vi "TEST_Camera_v2.vi"() -> ()   [LabVIEW 2018]
uses:
  <vilib>/vision/Image Controls.llb/IMAQ Image.ctl
  <vilib>/myRIO/Instrument Drivers/Onboard IO/PWM/PWM.lvlib
  <vilib>/vision/driver/NI_Vision_Acquisition_Software.lvlib
  <vilib>/vision/NI_Vision_Development_Module.lvlib
  <vilib>/myRIO/Instrument Drivers/Utilities/Utilities.lvlib
  <vilib>/myRIO/Instrument Drivers/Onboard IO/DIO/DIO.lvlib
  <vilib>/myRIO/Instrument Drivers/Onboard IO/PWM/typedefs/PWM Configuration.ctl
  <vilib>/myRIO/Common/Instrument Driver Framework/myRIO v1.0/PWM/typedefs/PWM Channels Enum.ctl
  <vilib>/myRIO/Common/Instrument Driver Framework/Utilities/typedefs/Generic FPGA Reference.ctl
  <vilib>/myRIO/Common/Instrument Driver Framework/Utilities/typedefs/myRIO v1.0 Reference.ctl
  <vilib>/myRIO/Common/Instrument Driver Framework/Utilities/typedefs/Hardware Version Enum.ctl
  <vilib>/myRIO/Common/Instrument Driver Framework/Utilities/typedefs/myRIO Generic Hardware Reference.ctl
  <vilib>/myRIO/Instrument Drivers/Onboard IO/PWM/typedefs/PWM Reference.ctl
  <vilib>/myRIO/Instrument Drivers/Onboard IO/PWM/vis/myRIO PWM Open.xnode
  <vilib>/myRIO/Common/Instrument Driver Framework/myRIO v1.0/PWM/vis/myRIO v1.1 Open PWM.vi
  <vilib>/userdefined/High Color/nirio_resource_hc.ctl
  <vilib>/myRIO/Instrument Drivers/Onboard IO/UART/typedef/VISA Configuration.ctl
  <vilib>/myRIO/Instrument Drivers/Onboard IO/UART/UART.lvlib
  <vilib>/Instr/_visa.llb/VISA Configure Serial Port (Instr).vi
panel:
  out "error out":errorcluster
  in  "error in (no error)":errorcluster
  out "Character Count":u32
  out "Image 7":T1(plugin-control)
  out "Image Pixels (U8)":u8[][](array[numeric])
  out "Image 6":T1(plugin-control)
  in  "Stop":bool
  out "Image 5":T1(plugin-control)
  out "Y":dbl[](array[numeric])
  out "X":dbl[](array[numeric])
  out "Antal isbjerg":i32
  out "logfile name":path
  in  "logfile base name":string="logfile"
  in  "Color Plane (Color Plane Extraction 1)":i32(ring)=1 items=["Red", "Green", "Blue", "Hue", "Saturation", "Luminance", "Value", "Intensity"]
  in  "Range (Threshold 1)":cluster{"Lower value":sgl, "Upper value":sgl}={"Lower value"=230.0, "Upper value"=255.0}
  in  "Structuring Element (Basic Morphology 1)":i32[][](array[numeric])=[[0, 1, 0], [1, 1, 1], [0, 1, 0]]
  in  "Number of Erosion (Advanced Morphology 1)":i32=12
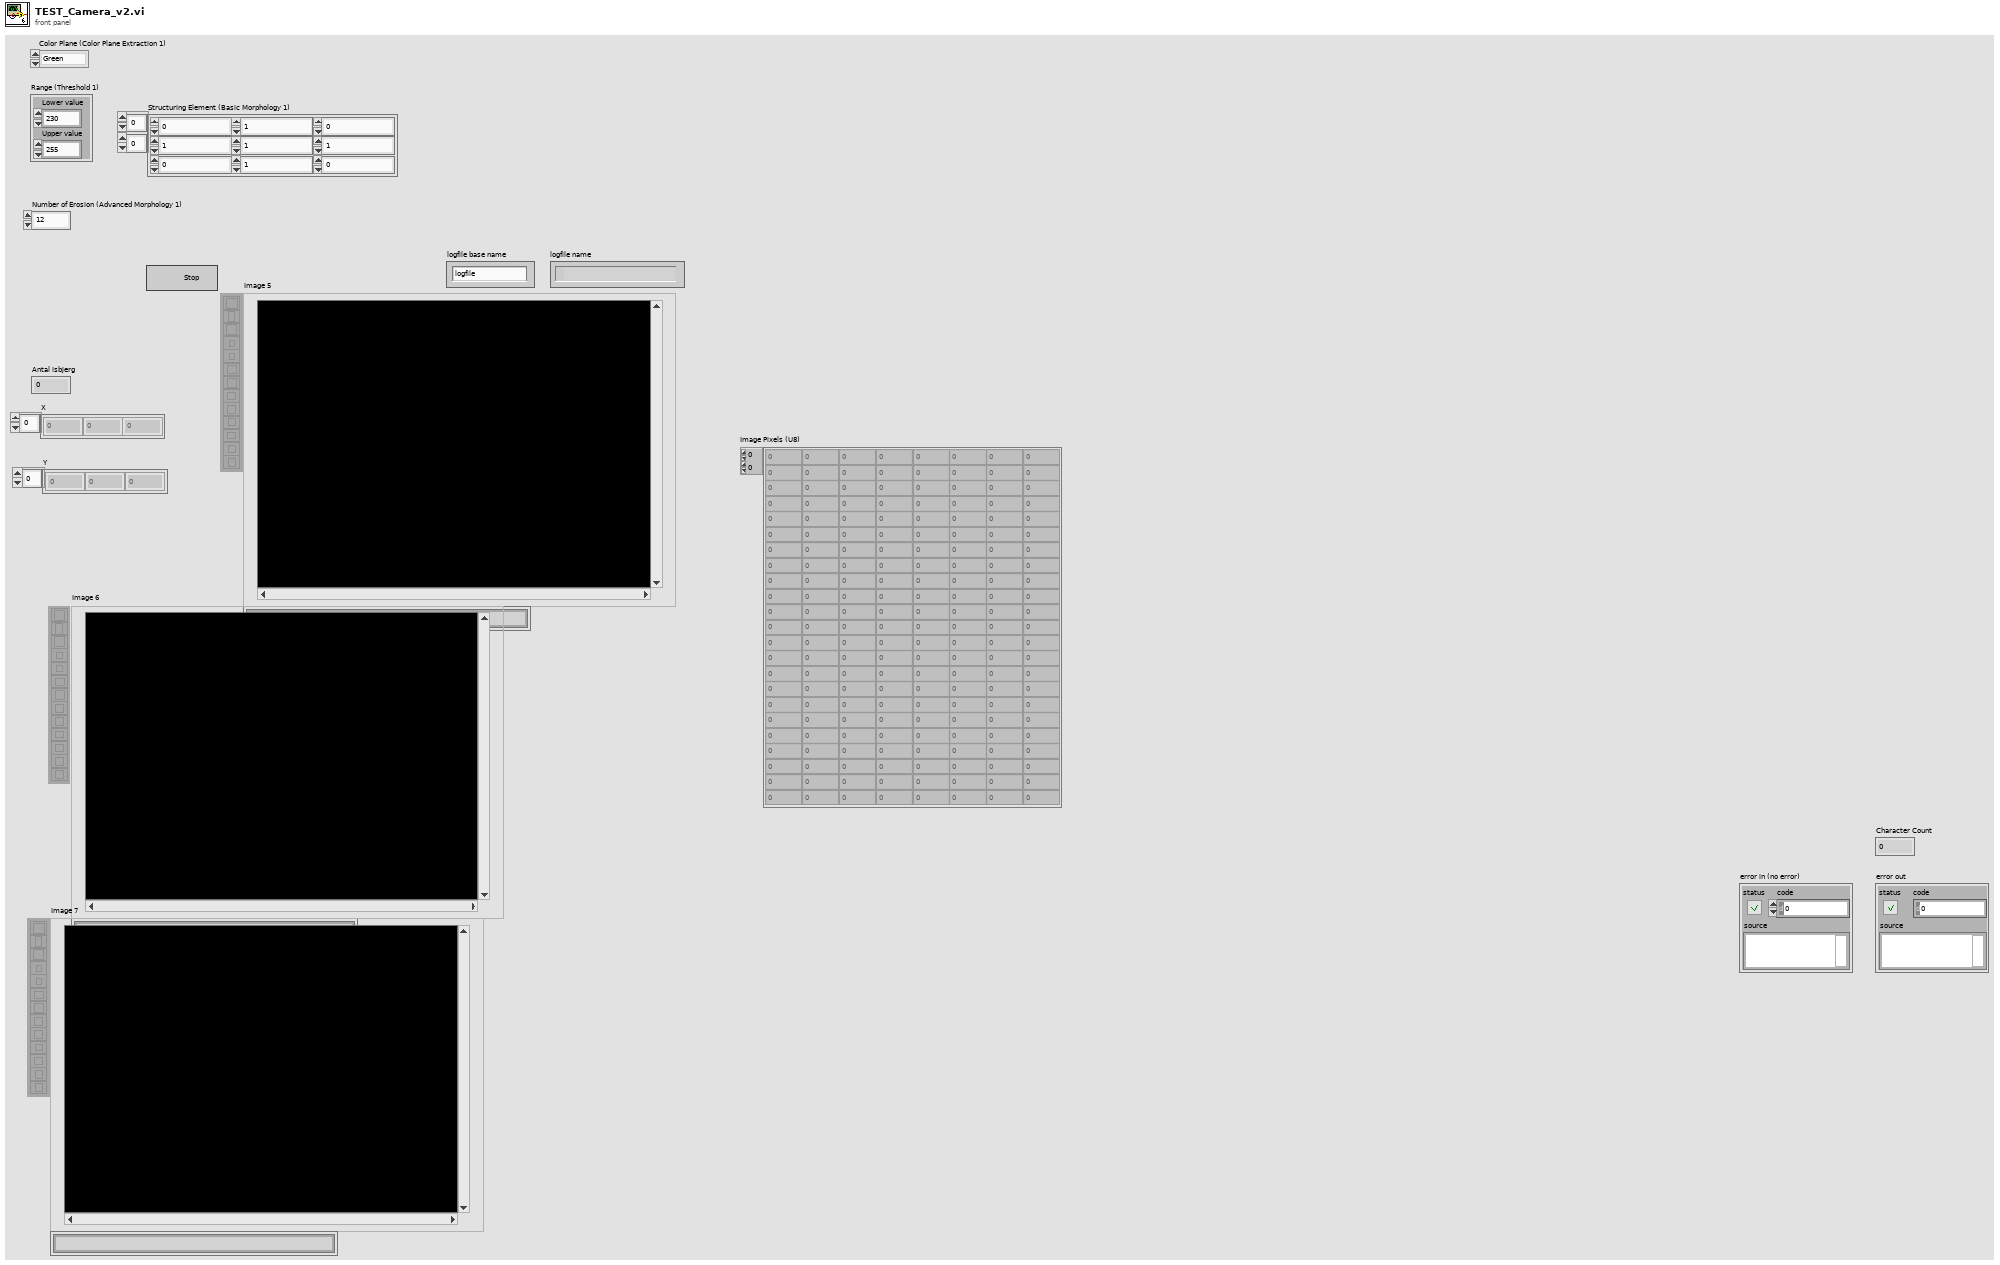
[diagram p1: front panel]
types:
  T1 = typedef "IMAQ Image.ctl" = refnum<image>
  T2 = typedef "UART.lvlib/VISA Configuration.ctl" = cluster{"baud rate (9600)":u32, "data bits (8)":u16, "parity (0:none)":enum16{"None", "Odd", "Even", "Mark", "Space"}, "stop bits (10: 1 bit)":u16, "flow control (0:none)":u16, "termination char\n(0xA = '\\n' = LF) ":u8, "Enable Termination\nChar (T)":bool, "timeout (10sec)":u32}
  T3 = typedef "PWM.lvlib/PWM Reference.ctl" = cluster{"myRIO Reference":T4, "PWM Channels Enum":T8, "PWM Configuration":T9}
  T4 = typedef "myRIO Generic Hardware Reference.ctl" = cluster{"myRIO Model":T5, "myRIO Hardware Reference":T6}
  T5 = typedef "Hardware Version Enum.ctl" = enum16{"Unknown", "myRIO-1900", "myRIO-1950", "roboRIO", "NI ELVIS RIO CM", "ELVIS III"}
  T6 = typedef "myRIO v1.0 Reference.ctl" = cluster{"Generic FPGA Reference":T7, "Allow multiple opens":bool}
  T7 = typedef "Generic FPGA Reference.ctl" = refnum<k20>
  T8 = typedef "PWM Channels Enum.ctl" = enum16{"Not Connected", "C/PWM0", "C/PWM1", "A/PWM0", "A/PWM1", "A/PWM2", "A/PWM3", "A/PWM4", "A/PWM5", "A/PWM6", "A/PWM7", "A/PWM8", "A/PWM9", "A/PWM10", "A/PWM11", "A/PWM12", "A/PWM13", "A/PWM14", "A/PWM15", "A/PWM16", "A/PWM17", "A/PWM18", "A/PWM19", "B/PWM0", "B/PWM1", "B/PWM2", "B/PWM3", "B/PWM4", "B/PWM5", "B/PWM6", "B/PWM7", "B/PWM8", "B/PWM9", "B/PWM10", "B/PWM11", "B/PWM12", "B/PWM13", "B/PWM14", "B/PWM15", "B/PWM16", "B/PWM17", "B/PWM18", "B/PWM19", "PWM/PWM0", "PWM/PWM1", "PWM/PWM2", "PWM/PWM3", "PWM/PWM4", "PWM/PWM5", "PWM/PWM6", "PWM/PWM7", "PWM/PWM8", "PWM/PWM9"}
  T9 = typedef "PWM.lvlib/PWM Configuration.ctl" = cluster{"Frequency":dbl, "Duty Cycle":dbl}
  T10 = enum32{"AutoM", "Close", "Dilate", "Erode", "Gradient", "Gradient out", "Gradient in", "Hit miss", "Open", "PClose", "POpen", "Thick", "Thin"}
  T11 = typedef "Image Type" = u32
  T12 = typedef "IMAQdx.ctl" = refnum<k21>
  T13 = typedef "DIO.lvlib/DIO Reference.ctl" = cluster{"myRIO Reference":T4, "DIO Channels List":T14}
  T14 = typedef "DIO Channels List.ctl" = T15[]
  T15 = typedef "DIO Channels Enum.ctl" = enum16{"Not Connected", "C/DIO0", "C/DIO1", "C/DIO2", "C/DIO3", "C/DIO4", "C/DIO5", "C/DIO6", "C/DIO7", "A/DIO0", "A/DIO1", "A/DIO2", "A/DIO3", "A/DIO4", "A/DIO5", "A/DIO6", "A/DIO7", "A/DIO8", "A/DIO9", "A/DIO10", "A/DIO11", "A/DIO12", "A/DIO13", "A/DIO14", "A/DIO15", "A/DIO16", "A/DIO17", "A/DIO18", "A/DIO19", "B/DIO0", "B/DIO1", "B/DIO2", "B/DIO3", "B/DIO4", "B/DIO5", "B/DIO6", "B/DIO7", "B/DIO8", "B/DIO9", "B/DIO10", "B/DIO11", "B/DIO12", "B/DIO13", "B/DIO14", "B/DIO15", "B/DIO16", "B/DIO17", "B/DIO18", "B/DIO19", "LED0", "LED1", "LED2", "LED3", "Button0", "DIO/DIO0", "DIO/DIO1", "DIO/DIO2", "DIO/DIO3", "DIO/DIO4", "DIO/DIO5", "DIO/DIO6", "DIO/DIO7", "DIO/DIO8", "DIO/DIO9", "SPI/CS0", "SPI/CS1", "SPI/CS2", "SPI/CS3", "LED RADIO (Green)", "LED RADIO (Red)", "LED COMM (Green)", "LED COMM (Red)", "LED MODE (Green)", "LED MODE (Red)"}
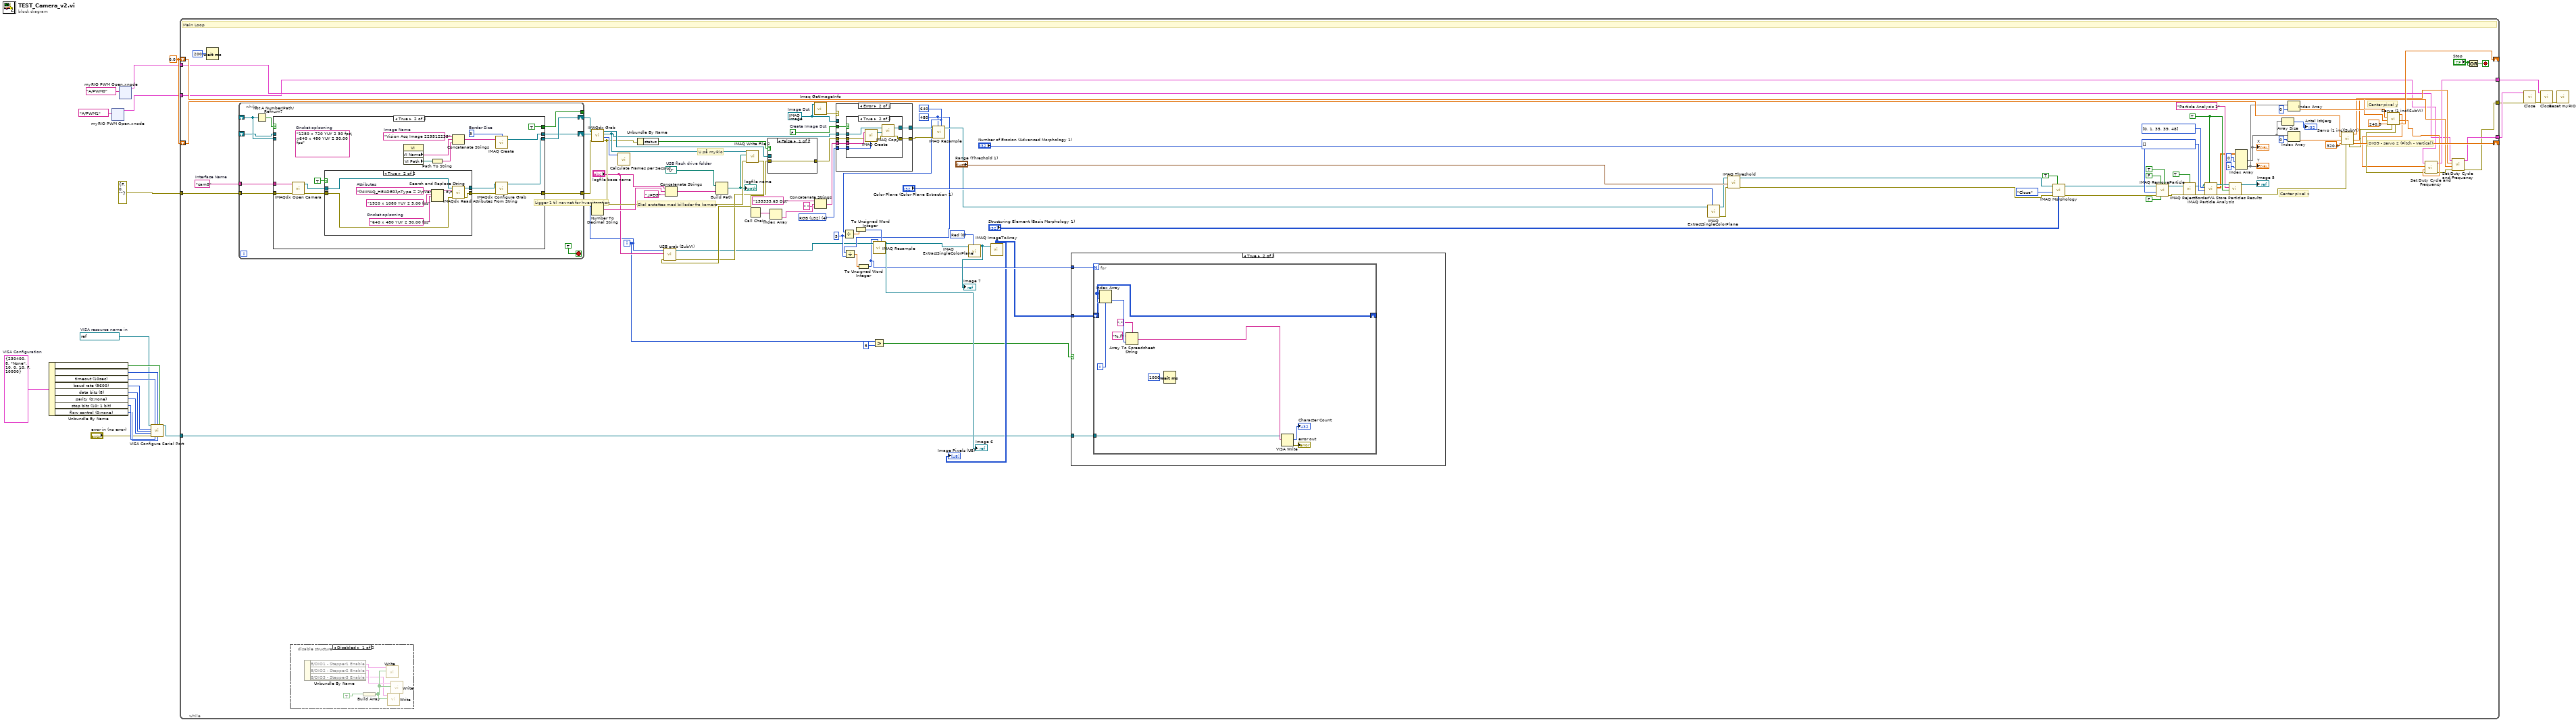
[diagram p0: block diagram]
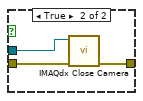
[diagram p4: hidden frame]
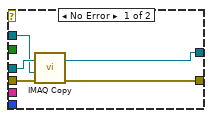
[diagram p7: hidden frame]
diagram:
  w3 = T2 {"baud rate (9600)"=230400, "data bits (8)"=8, "parity (0:none)"=enum."None", "stop bits (10: 1 bit)"=10, "flow control (0:none)"=0, "termination char\n(0xA = '\\n' = LF) "=10, "Enable Termination\nChar (T)"=FALSE, "timeout (10sec)"=10000}  # VISA Configuration
  w2 = refnum<visa-resource-name> "ASRL2::INSTR"  # VISA resource name in
  w22 = 0.0 ("Position 2")
  n1 = Unbundle By Name(w3) -> ("Enable Termination\nChar (T)"=w5:bool, "termination char\n(0xA = '\\n' = LF)"=w6:u8, "timeout (10sec)"=w7:u32, "baud rate (9600)"=w12:u32, "data bits (8)"=w11:u16, "parity (0:none)"=w10:enum16{"None", "Odd", "Even", "Mark", "Space"}, "stop bits (10: 1 bit)"=w9:u16, "flow control (0:none)"=w8:u16)
  n2 = xnode "myRIO PWM Open.xnode"("Channel Name"=tag "A/PWM1") -> ("PWM Ref Out"=w18:T3)  [unwired: 2 in, 1 out]
  n3 = xnode "myRIO PWM Open.xnode"("Channel Name"=tag "A/PWM0") -> ("PWM Ref Out"=w20:T3)  [unwired: 2 in, 1 out]
  n4 = call-poly "VISA Configure Serial Port"("VISA resource name"=w2, "timeout (10sec)"=w7, "termination char\n(0xA = '\\n' = LF)"=w6, "Enable Termination\nChar (T)"=w5, "baud rate (9600)"=w12, "data bits (8)"=w11, "parity (0:none)"=w10, "error in (no error)"="error in (no error)", "stop bits (10: 1 bit)"=w9, "flow control (0:none)"=w8) -> ("VISA resource name out"=w1:refnum<visa-resource-name>)  [unwired: 4 in, 1 out]
  n5 = while {
    shift-right: [w95] -> _
    shift-left: w22 -> [w98]
    shift-right: [w110] -> _
    shift-left: w22 -> [w111]
    tunnel: errorcluster {"status"=FALSE, "code"=0, "source"=""} ("error out") -> [w112]
    tunnel: [w48] -> w15
    tunnel: [w52] -> w16
    tunnel: [w51] -> w17
    tunnel: w20 -> [w31]
    tunnel: w18 -> [w30]
    tunnel: w1 -> [w27]
    i -> [w25]
    stop <- w129 stop-if-true
    w45 = 0 items=["Red", "Green", "Blue", "Hue", "Saturation", "Luminance", "Value", "Intensity"] ("Color Plane")
    w46 = u16 5 ("y")
    w40 = u32 640 ("Width")
    w39 = u32 480 ("Height")
    w67 = i32[] [] items=["Center of Mass X", "Center of Mass Y", "First Pixel X", "First Pixel Y", "Bounding Rect Left", "Bounding Rect Top", "Bounding Rect Right", "Bounding Rect Bottom", "Max Feret Diameter Start X", "Max Feret Diameter Start Y", "Max Feret Diameter End X", "Max Feret Diameter End Y", "Max Horiz. Segment Length Left", "Max Horiz. Segment Length Right", "Max Horiz. Segment Length Row", "-", "Bounding Rect Width", "Bounding Rect Height", "Bounding Rect Diagonal", "Perimeter", "Convex Hull Perimeter", "Holes' Perimeter", "Max Feret Diameter", "Equivalent Ellipse Major Axis", "Equivalent Ellipse Minor Axis", "Equivalent Ellipse Minor Axis (Feret)", "Equivalent Rect Long Side", "Equivalent Rect Short Side", "Equivalent Rect Diagonal", "Equivalent Rect Short Side (Feret)", "Average Horiz. Segment Length", "Average Vert. Segment Length", "Hydraulic Radius", "Waddel Disk Diameter", "-", "Area", "Holes' Area", "Particle & Holes' Area", "Convex Hull Area", "Image Area", "-", "Number of Holes", "Number of Horiz. Segments", "Number of Vert. Segments", "-", "Orientation", "Max Feret Diameter Orientation", "-", "% Area/Image Area", "% Area/(Particle & Holes' Area)", "Ratio of Equivalent Ellipse Axes", "Ratio of Equivalent Rect Sides", "-", "Elongation Factor", "Compactness Factor", "Heywood Circularity Factor", "Type Factor", "-", "Sum X", "Sum Y", "Sum XX", "Sum XY", "Sum YY", "Sum XXX", "Sum XXY", "Sum XYY", "Sum YYY", "-", "Moment of Inertia XX", "Moment of Inertia XY", "Moment of Inertia YY", "Moment of Inertia XXX", "Moment of Inertia XXY", "Moment of Inertia XYY", "Moment of Inertia YYY", "Norm. Moment of Inertia XX", "Norm. Moment of Inertia XY", "Norm. Moment of Inertia YY", "Norm. Moment of Inertia XXX", "Norm. Moment of Inertia XXY", "Norm. Moment of Inertia XYY", "Norm. Moment of Inertia YYY", "Hu Moment 1", "Hu Moment 2", "Hu Moment 3", "Hu Moment 4", "Hu Moment 5", "Hu Moment 6", "Hu Moment 7"] ("Real-World Measurements")
    w68 = i32[] [0, 1, 35, 39, 48] items=["Center of Mass X", "Center of Mass Y", "First Pixel X", "First Pixel Y", "Bounding Rect Left", "Bounding Rect Top", "Bounding Rect Right", "Bounding Rect Bottom", "Max Feret Diameter Start X", "Max Feret Diameter Start Y", "Max Feret Diameter End X", "Max Feret Diameter End Y", "Max Horiz. Segment Length Left", "Max Horiz. Segment Length Right", "Max Horiz. Segment Length Row", "-", "Bounding Rect Width", "Bounding Rect Height", "Bounding Rect Diagonal", "Perimeter", "Convex Hull Perimeter", "Holes' Perimeter", "Max Feret Diameter", "Equivalent Ellipse Major Axis", "Equivalent Ellipse Minor Axis", "Equivalent Ellipse Minor Axis (Feret)", "Equivalent Rect Long Side", "Equivalent Rect Short Side", "Equivalent Rect Diagonal", "Equivalent Rect Short Side (Feret)", "Average Horiz. Segment Length", "Average Vert. Segment Length", "Hydraulic Radius", "Waddel Disk Diameter", "-", "Area", "Holes' Area", "Particle & Holes' Area", "Convex Hull Area", "Image Area", "-", "Number of Holes", "Number of Horiz. Segments", "Number of Vert. Segments", "-", "Orientation", "Max Feret Diameter Orientation", "-", "% Area/Image Area", "% Area/(Particle & Holes' Area)", "Ratio of Equivalent Ellipse Axes", "Ratio of Equivalent Rect Sides", "-", "Elongation Factor", "Compactness Factor", "Heywood Circularity Factor", "Type Factor", "-", "Sum X", "Sum Y", "Sum XX", "Sum XY", "Sum YY", "Sum XXX", "Sum XXY", "Sum XYY", "Sum YYY", "-", "Moment of Inertia XX", "Moment of Inertia XY", "Moment of Inertia YY", "Moment of Inertia XXX", "Moment of Inertia XXY", "Moment of Inertia XYY", "Moment of Inertia YYY", "Norm. Moment of Inertia XX", "Norm. Moment of Inertia XY", "Norm. Moment of Inertia YY", "Norm. Moment of Inertia XXX", "Norm. Moment of Inertia XXY", "Norm. Moment of Inertia XYY", "Norm. Moment of Inertia YYY", "Hu Moment 1", "Hu Moment 2", "Hu Moment 3", "Hu Moment 4", "Hu Moment 5", "Hu Moment 6", "Hu Moment 7"] ("Pixel Measurements")
    w65 = TRUE ("Connectivity 4/8 (8)")
    w88 = path "U:/"  # USB flash drive folder
    w118 = "cam0"  # Interface Name
    w128 = T1 refnum  # Image Dst
    w120 = T11 4 items=["Grayscale (U8)", "Grayscale (I16)", "Grayscale (SGL)", "Complex (CSG)", "RGB (U32)", "HSL (U32)", "RGB (U64)", "Grayscale (U16)"] ("Image Dst Type")
    w126 = FALSE  # Create Image Dst
    # "U på myRio"
    # "Ligger 1 til navnet for hver iteration"
    # "Skal erstattes med billeder fra kamera"
    # "Center pixel y"
    # "Center pixel x"
    # "DIO9 - servo 2 (Pitch - Vertical)"
    # "Main Loop"
    n6 = Wait (ms)(milliseconds to wait=u32 200) -> ()  [unwired: 1 out]
    n7 = while "While Loop_template0" {
      shift-right: [w161] -> w113
      shift-left: _ -> [w154]
      tunnel: [w160] -> w119
      tunnel: w112 -> [w159]
      shift-right: [w157] -> w114
      shift-left: _ -> [w156]
      tunnel: w118 -> [w155]
      tunnel: [w152] -> _
      stop <- TRUE ("_template0") stop-if-true
      n8 = Not A Number/Path/Refnum?(number/path/refnum=w154) -> (NaN/Path/Refnum?=w153:bool)
      n9 = case "Case Structure_template0" shown="True" w153 {
        tunnel: [w164 w180] -> w161
        tunnel: w154 -> [w164 _]
        tunnel: [w163 w179] -> w160
        tunnel: w159 -> [w163 w181]
        tunnel: [w162 w178] -> w157
        tunnel: w156 -> [w162 _]
        tunnel: w155 -> [_ w169]
        tunnel: [_ TRUE] -> w152
        frame False {
        }
        frame True {
          (unwired) "1280 x 720 YUY 2 30 fps\n640 x 480 YUY 2 30.00 fps"  # Ønsket opløsning
          w166 = 3  # Border Size
          w173 = "Vision Acq Image 229512235"  # Image Name
          n10 = call <vilib>:"IMAQdx Open Camera.vi"("error in"=w181, "Session In"=w169) -> ("error out"=w171:errorcluster, "Session Out"=w172:T12)  [unwired: 1 in, 7 out]
          n11 = case shown="True" TRUE ("Init Attributes") {
            tunnel: w172 -> [w183 w191]
            tunnel: w171 -> [w182 w190]
            tunnel: [w183 w189] -> w165
            tunnel: [w182 w188] -> w170
            frame False {
            }
            frame True {
              w184 = "640 x 480 YUY 2 30.00 fps"  # Ønsket opløsning
              w187 = "[NIIMAQ_HEADER]\nType = 2\nVersion = 8\n\n[CAMERA_DATA]\nAcquisitionAttributes::Bayer::Algorithm = \"Bilinear\"\nAcquisitionAttributes::Bayer::GainB = \"1\"\nAcquisitionAttributes::Bayer::GainG = \"1\"\nAcquisitionAttributes::Bayer::GainR = \"1\"\nAcquisitionAttributes::Bayer::Pattern = \"Use hardware value\"\nAcquisitionAttributes::BitsPerPixel = \"Use hardware value\"\nAcquisitionAttributes::HardwareMaximumQueuedBufferCount = \"1000\"\nAcquisitionAttributes::HardwareRequeueBufferListThreshold = \"50\"\nAcquisitionAttributes::IgnoreFirstFrame = \"false\"\nAcquisitionAttributes::ImageDecoderCopyMode = \"Auto\"\nAcquisitionAttributes::OutputImageType = \"Auto\"\nAcquisitionAttributes::OverwriteMode = \"Get Newest\"\nAcquisitionAttributes::PixelSignedness = \"Use hardware value\"\nAcquisitionAttributes::ReceiveTimestampMode = \"None\"\nAcquisitionAttributes::ShiftPixelBits = \"false\"\nAcquisitionAttributes::SwapPixelBytes = \"false\"\nAcquisitionAttributes::Timeout = \"5000\"\nAcquisitionAttributes::VideoMode = \"1920 x 1080 YUY 2 5.00 fps\"\nCameraAttributes::BacklightCompensation::Mode = \"Manual\"\nCameraAttributes::BacklightCompensation::Value = \"0\"\nCameraAttributes::Brightness::Mode = \"Manual\"\nCameraAttributes::Brightness::Value = \"168\"\nCameraAttributes::Contrast::Mode = \"Manual\"\nCameraAttributes::Contrast::Value = \"5\"\nCameraAttributes::Exposure::Mode = \"AutoAperaturePriority\"\nCameraAttributes::Focus::Mode = \"Auto\"\nCameraAttributes::Pan::Mode = \"Manual\"\nCameraAttributes::Pan::Value = \"0\"\nCameraAttributes::PowerLineFrequency::Mode = \"60Hz\"\nCameraAttributes::Saturation::Mode = \"Manual\"\nCameraAttributes::Saturation::Value = \"103\"\nCameraAttributes::Sharpness::Mode = \"Manual\"\nCameraAttributes::Sharpness::Value = \"25\"\nCameraAttributes::Tilt::Mode = \"Manual\"\nCameraAttributes::Tilt::Value = \"0\"\nCameraAttributes::WhiteBalance::Mode = \"Auto\"\nCameraAttributes::Zoom::Mode = \"Manual\"\nCameraAttributes::Zoom::Value = \"0\"\n"  # Attributes
              n12 = Search and Replace String(input string=w187, search string="1920 x 1080 YUY 2 5.00 fps", replace string=w184) -> (result string=w185:string)  [unwired: 5 in, 3 out]
              n13 = call <vilib>:"IMAQdx Read Attributes From String.vi"("error in"=w190, "Attributes String In"=w185, "Session In"=w191) -> ("error out"=w188:errorcluster, "Session Out"=w189:T12)  [unwired: 7 out]
            }
          }
          n14 = property class="VI"() -> ("VI Name"=w176:string, "VI Path"=w177:path)  [unwired: 2 in, 2 out]
          n15 = Path To String(path=w177) -> (string=w175:string)
          n16 = Concatenate Strings(w173, w176, w175) -> (w174:string)
          n17 = call "IMAQ Create"("Border Size"=w166, "Image Name"=w174) -> ("New Image"=w178:T1)  [unwired: 2 in, 2 out]
          n18 = call <vilib>:"IMAQdx Configure Grab.vi"("error in"=w170, "Session In"=w165) -> ("error out"=w179:errorcluster, "Session Out"=w180:T12)  [unwired: 8 out]
        }
      }
    }
    n19 = disable-structure shown="Disabled" {
      frame Disabled {
        n20 = Unbundle By Name() -> ("B/DIO1 - Stepper1 Enable"=w145:T13, "B/DIO2 - Stepper2 Enable"=w144:T13, "B/DIO3 - Stepper3 Enable"=w143:T13)  [unwired: 1 in]
        n21 = Build Array(TRUE) -> (w146:bool[])
        n22 = call <vilib>:"Write.vi"("Values"=w146, "DIO Ref In"=w145) -> ()  [unwired: 7 in, 2 out]
        n23 = call <vilib>:"Write.vi"("Values"=w146, "DIO Ref In"=w143) -> ()  [unwired: 7 in, 2 out]
        n24 = call <vilib>:"Write.vi"("Values"=w146, "DIO Ref In"=w144) -> ()  [unwired: 7 in, 2 out]
      }
      frame Enabled {
      }
    }
    n25 = Number To Decimal String(number=w25) -> (decimal integer string=w91:string)  [unwired: 1 in]
    n26 = call <vilib>:"IMAQdx Grab.vi"("error in"=w119, "Image In"=w114, "Session In"=w113) -> ("error out"=w89:errorcluster, "Buffer Number Out"=w117:u32, "Image Out"=w90:T1, "Session Out"=w116:T12)  [unwired: 1 in, 4 out]
    n27 = call <vilib>:"Calculate Frames per Second.vi"("Buffer Number"=w117) -> ()  [unwired: 2 in, 9 out]
    n28 = Unbundle By Name(w89) -> ("status"=w107:bool)
    n29 = Concatenate Strings "Concatenate Strings"("logfile base name", w91, ".JPEG" ("string")) -> (w36:string)
    n30 = Build Path(base path=w88, name or relative path=w36) -> (appended path=w93:path)
    "logfile name" <- w93
    n31 = call-poly "IMAQ Write File 2"("error in (no error)"=w89, "File Path"=w93, "Image"=w90) -> ("error out"=w34:errorcluster)  [unwired: 7 in, 1 out]
    n32 = call "USB grab (SubVI).vi"("error in (no error)"=w34, "logfile base name in"="logfile base name", "Numeric"=w25) -> ("error out"=w33:errorcluster, "Refnum out"=w32:T1)  [unwired: 7 in]
    n33 = Call Chain() -> (call chain=w125:string[])
    n34 = case "Case Structure_template1" shown="False" w107 {
      tunnel: [w148 w150] -> w115
      tunnel: w33 -> [w148 w151]
      tunnel: w116 -> [_ w149]
      frame False {
      }
      frame True {
        n35 = call <vilib>:"IMAQdx Close Camera.vi"("error in"=w151, "Session In"=w149) -> ("error out"=w150:errorcluster)  [unwired: 9 out]
      }
    }
    n36 = Index Array(array=w125) -> (element=w123:string)  [unwired: 1 in]
    n37 = call "Imaq GetImageInfo"("Image"=w128) -> ("error out"=w127:errorcluster)  [unwired: 1 in, 9 out]
    n38 = Concatenate Strings("155335,63 Dst" ("Image Dst Name"), " ", w123) -> (w121:string)
    n39 = case shown="Error" w127 {
      tunnel: [w196 w200] -> w58
      tunnel: [w195 w199] -> w57
      tunnel: w90 -> [w194 w201]
      tunnel: w115 -> [w193 w197]
      tunnel: w128 -> [w192 _]
      tunnel: w121 -> [_ w203]
      tunnel: w120 -> [_ w202]
      tunnel: w126 -> [_ w198]
      frame No Error {
        n40 = call "IMAQ Copy"("error in (no error)"=w193, "Image Dst"=w192, "Image Src"=w194) -> ("error out"=w195:errorcluster, "Image Dst Out"=w196:T1)  [unwired: 3 out]
      }
      frame Error {
        n41 = case shown="True" w198 {
          tunnel: w203 -> [_ w213]
          tunnel: w202 -> [_ w212]
          tunnel: w201 -> [w205 w210]
          tunnel: [w205 w209] -> w200
          tunnel: [w204 w208] -> w199
          tunnel: w197 -> [w204 w206]
          frame False {
          }
          frame True {
            n42 = call "IMAQ Create"("Image Name"=w213, "Image Type"=w212, "error in (no error)"=w206) -> ("New Image"=w211:T1, "error out"=w207:errorcluster)  [unwired: 1 in, 1 out]
            n43 = call "IMAQ Copy"("error in (no error)"=w207, "Image Dst"=w211, "Image Src"=w210) -> ("error out"=w208:errorcluster, "Image Dst Out"=w209:T1)  [unwired: 3 out]
          }
        }
      }
    }
    n44 = Divide(x=w40, y=w46) -> (x/y=w43:dbl)
    n45 = Divide(x=w39, y=w46) -> (x/y=w44:dbl)
    n46 = To Unsigned Word Integer(number=w43) -> (unsigned 16bit integer=w42:u16)
    n47 = To Unsigned Word Integer(number=w44) -> (unsigned 16bit integer=w29:u16)
    n48 = call "IMAQ Resample"("X Resolution"=w42, "Y Resolution"=w29, "Image Src"=w32) -> ("Image Dst Out"=w38:T1)  [unwired: 7 in, 1 out]
    "Image 6" <- w38
    n49 = Greater?(x=w25, y=5) -> (0:w26:bool)
    n50 = call "IMAQ Resample"("X Resolution"=w40, "Y Resolution"=w39, "error in (no error)"=w57, "Image Src"=w58) -> ("Image Dst Out"=w41:T1)  [unwired: 6 in, 1 out]
    n51 = call "IMAQ ExtractSingleColorPlane"("Color Plane"=w45, "Image Src"=w38) -> ("Image Dst Out"=w37:T1)  [unwired: 8 in, 1 out]
    "Image 7" <- w37
    n52 = call "IMAQ ImageToArray"("Image"=w37) -> ("Image Pixels (U8)"=w28:u8[][])  [unwired: 3 in, 4 out]
    "Image Pixels (U8)" <- w28
    n53 = case shown="True" w26 {
      tunnel: w29 -> [_ w132]
      tunnel: w28 -> [_ w131]
      tunnel: w27 -> [_ w130]
      frame False {
      }
      frame True {
        n54 = for {
          N: w132 -> [_]
          shift-right: [w141] -> _
          shift-left: w131 -> [w141]
          tunnel: w130 -> [w134]
          i -> [w142]
          n55 = Index Array(array=w141, index (row)=w142) -> (element=w140:u8[])  [unwired: 1 in]
          n56 = Array To Spreadsheet String(delimiter (Tab)=",", array=w140, 3:"%.f" ("format string")) -> (spreadsheet string=w135:string)
          n57 = Wait (ms)(milliseconds to wait=u32 1000) -> ()  [unwired: 1 out]
          n58 = VISA Write(VISA resource name=w134, write buffer=w135) -> (return count=→"Character Count":u32, error out=→"error out":errorcluster)  [unwired: 1 in, 1 out]
        }
      }
    }
    n59 = call "IMAQ ExtractSingleColorPlane"("Color Plane"="Color Plane (Color Plane Extraction 1)", "Image Src"=w41) -> ("error out"=w86:errorcluster, "Image Dst Out"=w84:T1)  [unwired: 2 in, 6 out]
    n60 = call "IMAQ Threshold"("error in (no error)"=w86, "Range"="Range (Threshold 1)", "Image Src"=w84) -> ("error out"=w83:errorcluster, "Image Dst Out"=w79:T1)  [unwired: 3 in, 4 out]
    n61 = call "IMAQ Morphology"("Structuring Element"="Structuring Element (Basic Morphology 1)", "Square/Hexa (Square)"=TRUE, "error in (no error)"=w83, "Operation"=T10."Close", "Image Src"=w79) -> ("error out"=w78:errorcluster, "Image Dst Out"=w73:T1)  [unwired: 2 in, 3 out]
    n62 = call "IMAQ RemoveParticle"("Connectivity 4/8 (8)"=TRUE, "Low Pass/High Pass (Low)"=FALSE, "Square/Hexa (Square)"=FALSE, "error in (no error)"=w78, "Number of Erosion"="Number of Erosion (Advanced Morphology 1)", "Image Src"=w73) -> ("error out"=w72:errorcluster, "Image Dst Out"=w70:T1)  [unwired: 1 in, 3 out]
    n63 = call "IMAQ RejectBorder"("error in (no error)"=w72, "Image Src"=w70, "Connectivity 4/8 (8)"=TRUE) -> ("error out"=w69:errorcluster, "Image Dst Out"=w66:T1)  [unwired: 1 in, 2 out]
    n64 = call "IMAQ Particle Analysis"("Connectivity 4/8 (8)"=w65, "error in (no error)"=w69, "Real-World Measurements"=w67, "Pixel Measurements"=w68, "Image"=w66) -> ("error out"=w62:errorcluster, "Particle Measurements (Pixels)"=w59:dbl[][], "Image Out (duplicate)"=w64:T1)  [unwired: 4 out]
    n65 = call <vilib>:"IVA Store Particles Results.vi"("error in (no error)"=w62, "Connectivity 4/8 (8)"=w65, "Step Name"="Particle Analysis 1", "Image in"=w64) -> ("error out"=w60:errorcluster, "Image dup"=→"Image 5":T1)  [unwired: 6 out]
    n66 = Index Array(array=w59, index (col) #1=0 ("index (col)"), index (col) #2=1 ("index (col)")) -> (element #1=w102:dbl[], element #2=w99:dbl[])  [unwired: 2 in]
    "Y" <- w99
    "X" <- w102
    n67 = Array Size(array=w102) -> (size(s)=→"Antal isbjerg":i32)
    n68 = Index Array(array=w99, index=0) -> (element=w94:dbl)
    n69 = Index Array(array=w102, index=0) -> (element=w101:dbl)
    n70 = call "Servo (1 inc)(SubVI).vi"("error constant 2"=w60, "Center pixel"=320.0 ("Center pixel 2"), "Pixel value"=w101, "Position."=w111) -> ("Position 2"=w110:dbl, "freq [Hz]"=w53:dbl, "Duty"=w54:dbl, "error constant"=w96:errorcluster)  [unwired: 3 in, 1 out]
    n71 = call "Servo (1 inc)(SubVI).vi"("error constant 2"=w96, "Center pixel"=240.0, "Pixel value"=w94, "Position."=w98) -> ("Position 2"=w95:dbl, "freq [Hz]"=w55:dbl, "Duty"=w47:dbl, "error constant"=w50:errorcluster)  [unwired: 3 in, 1 out]
    n72 = call <vilib>:"Set Duty Cycle and Frequency.vi"("error in (no error)"=w50, "Frequency [Hz]"=w55, "Duty Cycle"=w47, "PWM Ref In"=w30) -> ("error out"=w49:errorcluster, "PWM Ref Out"=w52:T3)  [unwired: 5 in]
    n73 = call <vilib>:"Set Duty Cycle and Frequency.vi"("error in (no error)"=w49, "Frequency [Hz]"=w53, "Duty Cycle"=w54, "PWM Ref In"=w31) -> ("error out"=w48:errorcluster, "PWM Ref Out"=w51:T3)  [unwired: 5 in]
    n74 = Or(x="Stop", y="Stop") -> (x .or. y?=w129:bool)
  }
  n75 = call <vilib>:"Close.vi"("error in (no error)"=w15, "PWM Ref In"=w17) -> ("error out"=w14:errorcluster)  [unwired: 9 in]
  n76 = call <vilib>:"Close.vi"("error in (no error)"=w14, "PWM Ref In"=w16) -> ("error out"=w13:errorcluster)  [unwired: 9 in]
  n77 = call <vilib>:"Reset myRIO.vi"("error in (no error)"=w13) -> ()  [unwired: 10 in, 1 out]
